vi "Send StopProcessedEvent.vi"(8 "error in (no error)":errorcluster, 11 "SMO":refnum<class "SMO.lvclass">) -> (0 "error out":errorcluster, 3 "SMO out":refnum<class "SMO.lvclass">)   [LabVIEW 2021, in "smo.lvlib" / "SMO.lvclass"]
uses:
  SMO.lvclass
  Typedefs/StopProcessEventData--Cluster.ctl
  SMO.lvclass/SMO.ctl
  ReftoDVR--SMO.vi
panel:
  # "For instructions on how to use the JKI State Machine Objects, examples and video tutorials, visit:\nhttp://jki.net/state-machine-objects/\n\nJKI State Machine Objects™\nhttp://jki.net/state-machine-objects/\nCopyright (C) 2005-2015, JKI <info@jki.net>\nALL RIGHTS RESERVED"
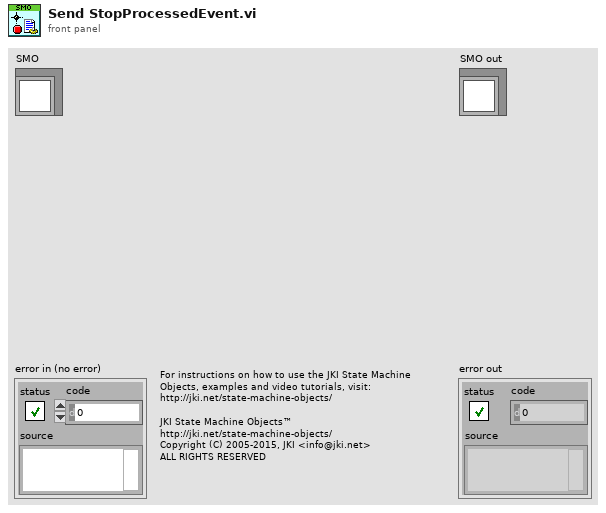
[diagram p1: front panel]
types:
  T1 = typedef "smo.lvlib/SMO.lvclass/StopProcessEventData--Cluster.ctl" = cluster{"Time Stamp":timestamp}
  T2 = typedef "smo.lvlib/SMO.lvclass/Protected Events.ctl" = cluster{"StopProcesses":refnum<user-event>, "AbortProcesses":refnum<user-event>, "Config Changed":refnum<user-event>, "Dependency":refnum<user-event>}
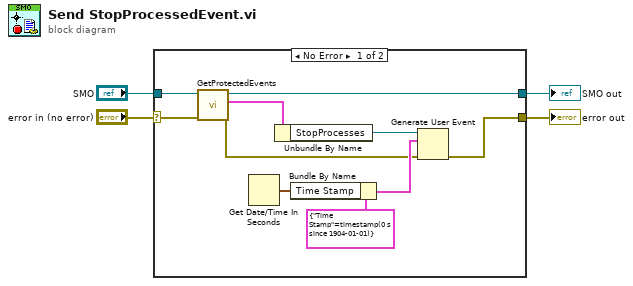
[diagram p0: block diagram]
diagram:
  n1 = case shown="No Error" "error in (no error)" {
    selector: "error in (no error)" -> [w5 w16]
    tunnel: [w11 w16] -> w3
    tunnel: [w8 w15] -> w1
    tunnel: "SMO" -> [w9 w15]
    frame No Error {
      n2 = call "GetProtectedEvents.vi"("error in (no error)"=w5, "SMO"=w9) -> ("error out"=w6:errorcluster, "SMO Protected Events"=w7:T2, "SMO out"=w8:refnum<class "SMO.lvclass">)  [unwired: 7 in]
      n3 = Get Date/Time In Seconds() -> (seconds since 1Jan1904=w13:timestamp)
      n4 = Unbundle By Name(w7) -> ("StopProcesses"=w12:refnum<user-event>)
      n5 = Bundle By Name(cluster=T1 {"Time Stamp"=timestamp(0 s since 1904-01-01)} ("Stop Processes Event Data"), "Time Stamp"=w13) -> (w14:T1)
      n6 = Generate User Event(user event=w12, event data cluster=w14, error in=w6) -> (error out=w11:errorcluster)  [unwired: 1 in, 1 out]
    }
    frame Error {
    }
  }
  "error out" <- w3
  "SMO out" <- w1
